vi "SetBusClass.vi"(8 "ErrorArray In":errorcluster[](array[cluster]), 11 "Framework.lvlib:Bus.lvclass":refnum<class "Bus.lvclass">) -> (0 "ErrorArray Out":errorcluster[](array[cluster]))   [LabVIEW 2014]
uses:
  Bus.lvclass
  Framework.lvlib
  <userlib>/NIST/NISTErrorLib/NISTErrorLib.lvlib
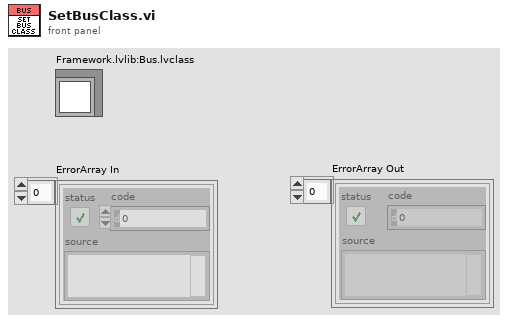
[diagram p1: front panel]
types:
  T1 = typedef "Framework.lvlib/clFrameworkData.ctl" = cluster{"EvtINIFilePaths":path[], "BusClassInstances":refnum<class "Bus.lvclass">[], "PmuImpairINIFilePaths":path[], "FlagImpairINIFilePaths":path[], "NetImpairINIFilePaths":path[], "OutputToFileINIFilePaths":path[], "AppINIFilePaths":path[], "AppModuleID":i32, "OutputToFileID":i32}
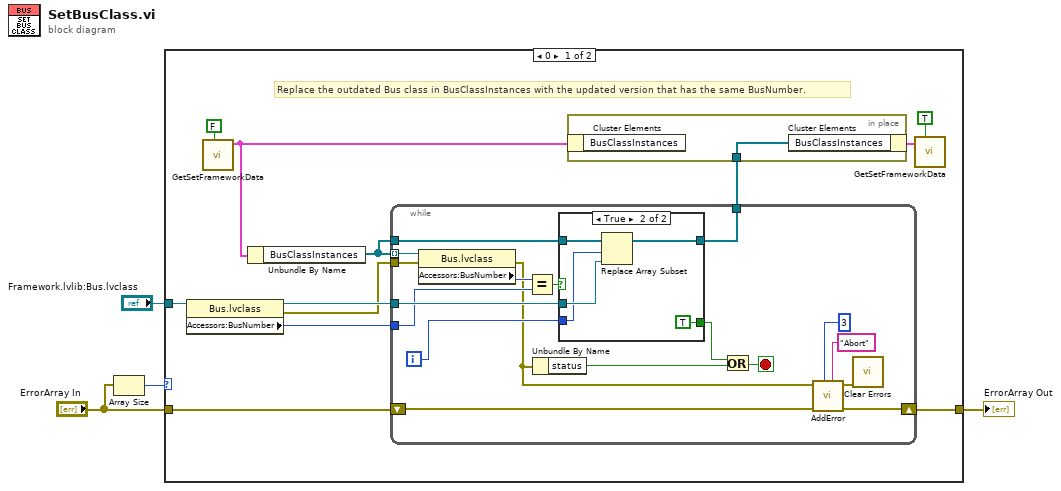
[diagram p0: block diagram]
diagram:
  n1 = Array Size(array="ErrorArray In") -> (size(s)=w4:i32)
  n2 = case shown="0" w4 {
    tunnel: "ErrorArray In" -> [w7 w42]
    tunnel: [w6 w42] -> w2
    tunnel: "Framework.lvlib:Bus.lvclass" -> [w16 _]
    frame 0 {
      # "Replace the outdated Bus class in BusClassInstances with the updated version that has the same BusNumber."
      n3 = property class="Bus.lvclass"(reference=w16) -> (reference out=w9:refnum<class "Bus.lvclass">, error out=w5:errorcluster, "Accessors:BusNumber"=w8:u8)  [unwired: 1 in]
      n4 = call "GetSetFrameworkData.vi"("Set (F)"=FALSE ("Set/Get")) -> ("clFrameworkData Out"=w12:T1)  [unwired: 10 in]
      n5 = Unbundle By Name(w12) -> ("BusClassInstances"=w14:refnum<class "Bus.lvclass">[])
      n6 = while {
        tunnel: w14 -> [w33] mode=indexing
        tunnel: w9 -> [w29]
        tunnel: w14 -> [w28]
        tunnel: [w26] -> w11
        tunnel: w8 -> [w25]
        shift-right: [w21] -> w6
        shift-left: w7 -> [w20]
        tunnel: w5 -> [w18]
        i -> [w27]
        stop <- w31 stop-if-true
        n7 = property class="Bus.lvclass"(reference=w33, error in=w18) -> (error out=w19:errorcluster, "Accessors:BusNumber"=w35:u8)  [unwired: 1 out]
        n8 = Equal?(x=w35, y=w25) -> (x = y?=w34:bool)
        n9 = Unbundle By Name(w19) -> ("status"=w32:bool)
        n10 = case shown="True" w34 {
          tunnel: [_ TRUE] -> w30
          tunnel: w29 -> [_ w39]
          tunnel: w28 -> [w36 w40]
          tunnel: w27 -> [_ w38]
          tunnel: [w36 w37] -> w26
          frame False {
          }
          frame True {
            n11 = Replace Array Subset(array=w40, new element=w39, index=w38) -> (w37:refnum<class "Bus.lvclass">[])
          }
        }
        n12 = Or(x=w30, y=w32) -> (x .or. y?=w31:bool)
        n13 = call <userlib>:"AddError.vi"("Severity"="Abort" ("String"), "Priority"=u8 3, "ErrorArray"=w20, "error in (no error)"=w19) -> ("ErrorArray"=w21:errorcluster[], "error out"=w24:errorcluster)  [unwired: 6 in]
        n14 = call <vilib>:"Clear Errors.vi"("error in (no error)"=w24) -> ()  [unwired: 5 in, 2 out]
      }
      n15 = in-place {
        in-place-border: w11 -> [w17]
        n16 = in-place-cluster #1(w12) -> ()  [unwired: 1 out]
        n17 = in-place-cluster #1("BusClassInstances"=w17) -> (w10:T1)
      }
      n18 = call "GetSetFrameworkData.vi"("Set (F)"=TRUE ("Set/Get"), "clFrameworkData In"=w10) -> ()  [unwired: 9 in, 1 out]
    }
    frame 1, Default {
      # "External error.  Error array holds at least one error."
    }
  }
  "ErrorArray Out" <- w2
